vi "EvaluateMotorLimits.vi"(0 "MotorMeasurements":T1, 1 "Commanded RPM":dbl, 2 "RPM Tolerance":dbl, 3 "Test Current Limit (A)":dbl, 4 "Test Temperature Limit (°C)":dbl, 5 "Test Vibration Limit (mm/s)":dbl, 6 "Safety Current Trip (A)":dbl, 7 "Safety Temperature Trip (°C)":dbl, 9 "Safety Vibration Trip (mm/s)":dbl) -> (16 "SYSTEM FAULT REQUEST":bool, 18 "CURRENT SAMPLE FAILED":bool, 20 "RPM OK":bool, 21 "CURRENT OK":bool, 22 "TEMPERATURE OK":bool, 23 "VIBRATION OK":bool, 24 "CURRENT TRIP":bool, 25 "TEMPERATURE TRIP":bool, 26 "VIBRATION TRIP":bool, 27 "RPM Error":dbl)   [LabVIEW 2026]
uses:
  MotorMeasurements.ctl
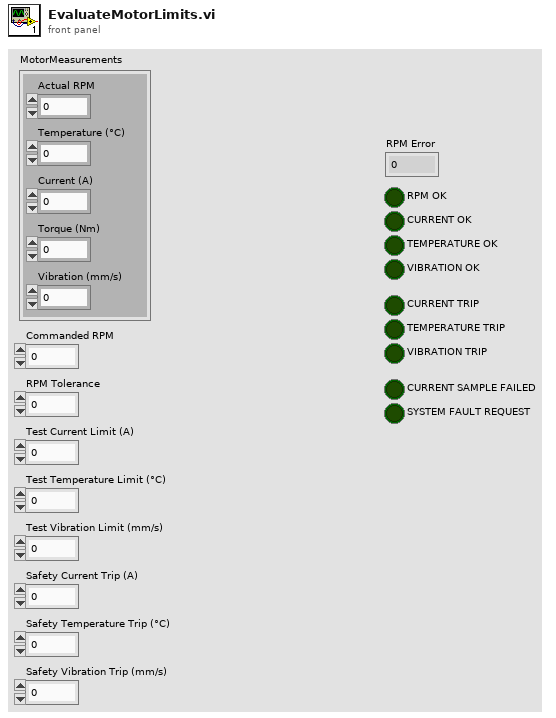
[diagram p1: front panel]
types:
  T1 = typedef "MotorMeasurements.ctl" = cluster{"Temperature (°C)":dbl, "Current (A)":dbl, "Torque (Nm)":dbl, "Vibration (mm/s)":dbl, "Actual RPM":dbl}
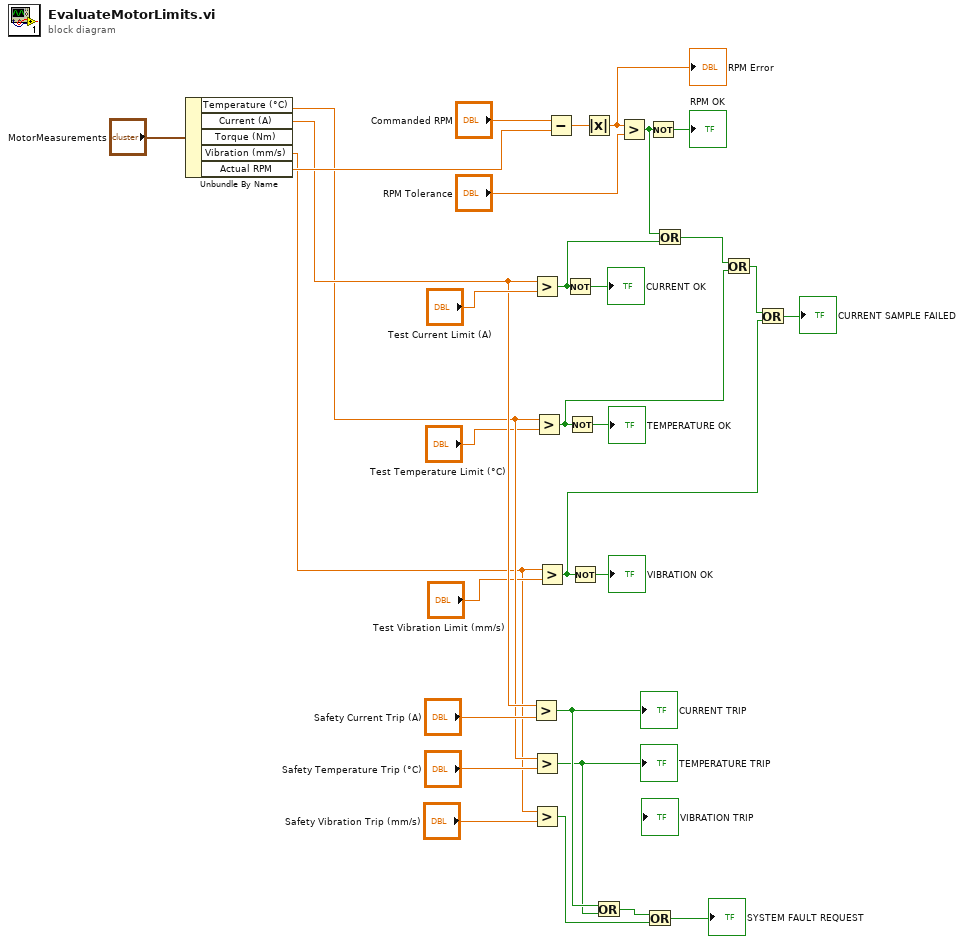
[diagram p0: block diagram]
diagram:
  n1 = Unbundle By Name("MotorMeasurements") -> ("Temperature (°C)"=w12:dbl, "Current (A)"=w13:dbl, "Vibration (mm/s)"=w1:dbl, "Actual RPM"=w14:dbl)  [unwired: 1 out]
  n2 = Greater?(x=w13, y="Safety Current Trip (A)") -> (0:w18:bool)
  "CURRENT TRIP" <- w18
  n3 = Greater?(x=w13, y="Test Current Limit (A)") -> (0:w23:bool)
  n4 = Greater?(x=w12, y="Safety Temperature Trip (°C)") -> (0:w17:bool)
  "TEMPERATURE TRIP" <- w17
  n5 = Greater?(x=w1, y="Safety Vibration Trip (mm/s)") -> (0:w9:bool)
  n6 = Greater?(x=w12, y="Test Temperature Limit (°C)") -> (0:w22:bool)
  n7 = Greater?(x=w1, y="Test Vibration Limit (mm/s)") -> (0:w4:bool)
  n8 = Subtract(x="Commanded RPM", y=w14) -> (x-y=w31:dbl)
  n9 = Not(x=w23) -> (.not. x?=→"CURRENT OK":bool)
  n10 = Not(x=w22) -> (.not. x?=→"TEMPERATURE OK":bool)
  n11 = Not(x=w4) -> (.not. x?=→"VIBRATION OK":bool)
  n12 = Absolute Value(x=w31) -> (abs(x)=w19:dbl)
  "RPM Error" <- w19
  n13 = Or(x=w18, y=w17) -> (x .or. y?=w10:bool)
  n14 = Greater?(x=w19, y="RPM Tolerance") -> (0:w24:bool)
  n15 = Or(x=w10, y=w9) -> (x .or. y?=→"SYSTEM FAULT REQUEST":bool)
  n16 = Not(x=w24) -> (.not. x?=→"RPM OK":bool)
  n17 = Or(x=w24, y=w23) -> (x .or. y?=w25:bool)
  n18 = Or(x=w25, y=w22) -> (x .or. y?=w3:bool)
  n19 = Or(x=w3, y=w4) -> (x .or. y?=→"CURRENT SAMPLE FAILED":bool)
